vi "Handle Last Ack Core.vi"(4 "error in (no error)":errorcluster, 6 "Last Ack":refnum<class "Last Ack.lvclass">, 7 "Caller Endpoint in":refnum<class "Caller Endpoint.lvclass">) -> (0 "error out":errorcluster, 3 "Caller Endpoint out":refnum<class "Caller Endpoint.lvclass">)   [LabVIEW 2020, in "Caller Endpoint.lvlib" / "Caller Endpoint.lvclass"]
doc: "(<B>Filename</B>: Actor Framework.lvlib:Actor.lvclass:Handle Last Ack Core.vi)\n\nDefines how the caller actor responds to the Last Ack message from a nested actor. The Last Ack message is the final message a nested actor sends to its caller before it shuts down. The message contains information about the final state of the nested actor.\n\nBy default, this method does nothing except return any error the nested actor sent. A descendant class may override this method to define behavior."
uses:
  <vilib>/NI/Actors/Network Endpoint Actors/Caller Endpoint/Caller Endpoint/Caller Endpoint.lvclass
  <vilib>/ActorFramework/LastAck/Last Ack.lvclass
  C:/Program Files (x86)/National Instruments/LabVIEW 2020/vi.lib/ActorFramework/Message/Message.lvclass
  C:/Program Files (x86)/National Instruments/LabVIEW 2020/vi.lib/NI/Actors/Network Endpoint Actors/Network Endpoint/Network Endpoint/Network Endpoint.lvclass
  <vilib>/NI/Actors/Network Endpoint Actors/Network Endpoint/Network Endpoint/Network Endpoint.lvclass/Network Endpoint.ctl
  <vilib>/NI/Actors/Network Endpoint Actors/Network Endpoint/Network Endpoint/Network Endpoint.lvclass
  <vilib>/NI/Actors/Network Endpoint Actors/Abstract Classes/Message Stream/Message Stream.lvclass
  <resource>/AFDebug/AF Debug.lvlib
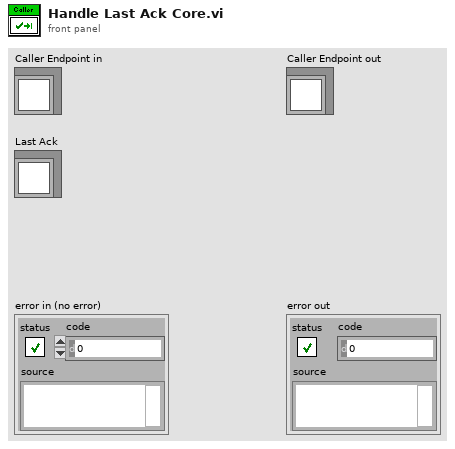
[diagram p1: front panel]
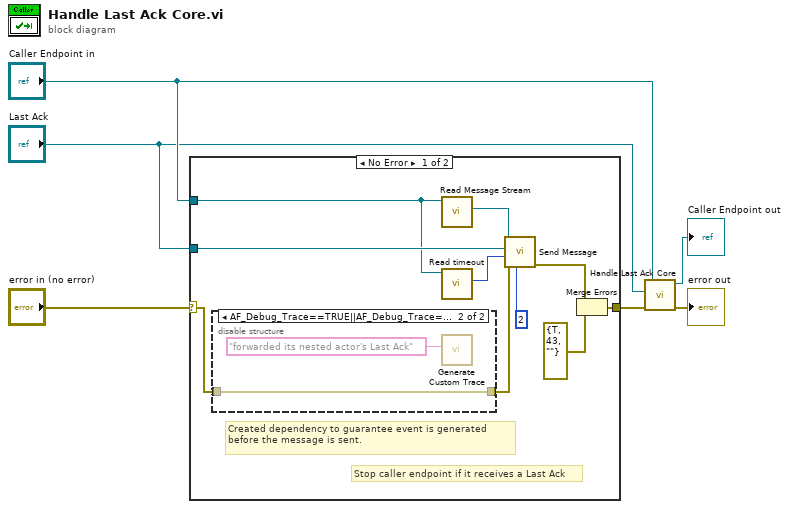
[diagram p0: block diagram]
diagram:
  n1 = case shown="No Error" "error in (no error)" {
    selector: "error in (no error)" -> [w11 w20]
    tunnel: "Last Ack" -> [w16 _]
    tunnel: "Caller Endpoint in" -> [w14 _]
    tunnel: [w9 w20] -> w3
    frame No Error {
      # "Stop caller endpoint if it receives a Last Ack"
      # "Created dependency to guarantee event is generated before the message is sent."
      n2 = disable-structure shown="AF_Debug_Trace==TRUE||AF_Debug_Trace==True" {
        disable-tunnel: w11 -> [w17 w18]
        disable-tunnel: [w17 w18] -> w10
        frame condition #0 (active) {
        }
        frame condition #1 {
          n3 = call <resource>:"Generate Custom Trace.vi"("Custom Action"="forwarded its nested actor's Last Ack" ("format string")) -> ()  [unwired: 11 in]
        }
      }
      n4 = call <vilib>:"Read Message Stream.vi"("Network Endpoint in"=w14) -> ("Message Stream"=w15:refnum<class "Message Stream.lvclass">)  [unwired: 10 in]
      n5 = call <vilib>:"Read timeout.vi"("Network Endpoint in"=w14) -> ("timeout"=w13:i32)  [unwired: 10 in]
      n6 = call-dynamic "Send Message.vi"("priority"=2, "error in (no error)"=w10, "timeout ms (-1)"=w13, "Message"=w16, "Message Stream in"=w15) -> ("error out"=w8:errorcluster)  [unwired: 5 in, 1 out]
      n7 = Merge Errors(w8, errorcluster {"status"=TRUE, "code"=43, "source"=""} ("error in")) -> (w9:errorcluster)
    }
    frame Error {
    }
  }
  n8 = call-parent "Handle Last Ack Core.vi"("error in (no error)"=w3, "Last Ack"="Last Ack", "Actor in"="Caller Endpoint in") -> ("error out"=→"error out":errorcluster, "Actor out"=→"Caller Endpoint out":refnum<class "Caller Endpoint.lvclass">)  [unwired: 3 in]
